vi "getInstanceCmd.vi"(8 "error in (no error)":errorcluster, 11 "tcpServer in":refnum<class "TcpServer.lvclass">) -> (0 "error out":errorcluster, 2 "CmdRead":refnum<user-event>, 3 "tcpServer out":refnum<class "TcpServer.lvclass">)   [LabVIEW 2018, in "TcpServer.lvclass"]
doc: "Get the CmdRead user event instance, to read commands from TCP Client."
uses:
  TcpServer.lvclass
  TcpServer.lvclass/TcpServer.ctl
  TcpServerCmd/TcpServerCmd.lvclass/TcpServerCmd.ctl
  TcpServerCmd/TcpServerCmd.lvclass
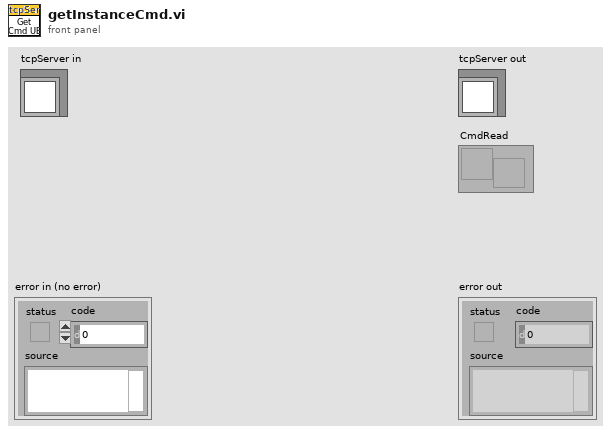
[diagram p1: front panel]
types:
  T1 = typedef "TcpServerCmd.lvclass/userEventTypeDef.ctl" = cluster{"CmdRead":refnum<user-event>, "CmdWrite":refnum<user-event>, "EvtRead":refnum<user-event>, "EvtWrite":refnum<user-event>, "GenRead":refnum<user-event>, "GenWrite":refnum<user-event>}
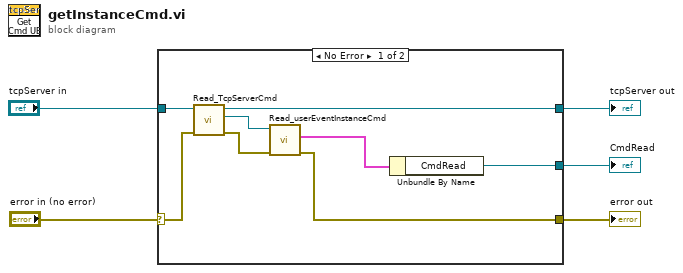
[diagram p0: block diagram]
diagram:
  n1 = case shown="No Error" "error in (no error)" {
    selector: "error in (no error)" -> [w6 w15]
    tunnel: [w9 w15] -> w4
    tunnel: [w10 w14] -> w2
    tunnel: "tcpServer in" -> [w13 w14]
    tunnel: [w12 _] -> w1
    frame No Error {
      n2 = call "Read_TcpServerCmd.vi"("error in (no error)"=w6, "TcpServer in"=w13) -> ("error out"=w7:errorcluster, "TcpServerCmd.lvclass"=w11:refnum<class "TcpServerCmd.lvclass">, "TcpServer out"=w10:refnum<class "TcpServer.lvclass">)  [unwired: 7 in]
      n3 = call "Read_userEventInstanceCmd.vi"("error in (no error)"=w7, "TcpServerCmd in"=w11) -> ("error out"=w9:errorcluster, "userEventInstance"=w8:T1)  [unwired: 7 in, 1 out]
      n4 = Unbundle By Name(w8) -> ("CmdRead"=w12:refnum<user-event>)
    }
    frame Error {
    }
  }
  "error out" <- w4
  "tcpServer out" <- w2
  "CmdRead" <- w1
